vi "SVT STFT vs Time (Intensity).vi"(0 "scaled signal [EU]":waveform(dbl), 5 "FFT block size":i32=1024 min=1, 7 "window":T8(ring)=enum."Hanning", 9 "time segment":T7={"from [s]"=-1.0, "to [s]"=-1.0, "time increment"=100.0, "time increment units (%)"=enum."%"} {"time increment" format="%.2f"; "to [s]" format="%.2f"; "from [s]" format="%.2f"}, 11 "error in (no error)":errorcluster, 12 "dB On (T)":bool=TRUE, 13 "weighting":u16(ring) items=["Linear", "A-weighting", "B-weighting", "C-weighting"]) -> (4 "power spectra [dB EU]":dbl[][](array[numeric]) format="%.2f", 6 "unit label":string, 8 "f0 and delta f [Hz]":cluster{"f0":dbl, "delta f":dbl}={"f0"=0.0, "delta f"=0.0009765625} {"delta f" format="%.2f"; "f0" format="%.2f"}, 10 "t0 and delta t [s]":cluster{"t0":dbl, "delta t":dbl} {"delta t" format="%.2f"; "t0" format="%.2f"}, 14 "spectrum info":T1={"channel name"="", "description"="", "x-axis units"=0, "spectral info"={"spectrum type"=enum."Power [Magnitude^2]", "linear/dB"=enum."linear", "window"=0, "window size"=0, "FFT size"=0}, "engineering units"=0, "custom label"="", "dB reference [EU]"=0.0, "peak units"=enum."rms", "weighting filter"=0, "spectral density?"=FALSE, "unit label"="", "spectrum skewed?"=FALSE, "complimentary spectrum units"=enum."none"} {"x-axis units" items=["Time (s)"=0, "Frequency-CB (Hz)"=1, "Frequency-CPB (Hz)"=1248, "Frequency-Arbitrary (Hz)"=2357, "Quefrency (s)"=2, "Revolutions (rev)"=3, "Order"=4, "Speed (RPM)"=11, "Speed (rad/s)"=21, "Index"=65535]; "weighting filter" items=["Linear", "A-weighting", "B-weighting", "C-weighting", "ITU-R 468-4", "Dolby", "CCITT", "C-message", "Wb", "Wc", "Wd", "We", "Wf", "Wh", "Wj", "Wk", "Wm", "AES17 20 kHz lowpass", "AES17 40 kHz lowpass", "AES17 20 kHz highpass", "AES17 40 kHz highpass"]; "dB reference [EU]" format="%.2f"; "engineering units" items=["custom..."=0, "V"=1, "A"=21, "C"=30, "pC"=31, "s"=32, "-"=29, "Pa"=2, "N"=20, "g"=3, "m/s^2"=4, "m/s"=5, "m"=6, "mm/s"=12, "mm"=13, "micron/s"=14, "micron"=15, "in/s^2"=7, "in/s"=8, "in"=9, "mil/s"=10, "mil"=11, "rad/s^2"=16, "rad/s"=17, "rad"=18, "deg/s^2"=26, "deg/s"=27, "deg"=28, "RPM"=22, "cycle/s^2"=23, "Hz"=24, "cycle"=25, "strain"=19]; "spectral info"."window" items=["None "=0, "Hanning"=1, "Hamming"=2, "Blackman-Harris"=3, "Exact Blackman"=4, "Blackman"=5, "Flat Top"=6, "4 Term B-Harris "=7, "7 Term B-Harris"=8, "Low Sidelobe"=9, "Force - Exponential"=10, "Gaussian"=62]}, 15 "error out":errorcluster)   [LabVIEW 2017, in "SoundVib_Transient.lvlib"]
doc: "Performs a short-time Fourier transform (STFT) on <B>scaled signal [EU]</B> and returns the power spectrum, waterfall, or colormap at the various times you specify. Wire data to the <B>scaled signal [EU]</B> input to determine the polymorphic instance to use or manually select the instance."
uses:
  <vilib>/addons/Sound and Vibration/svt_Transients/SoundVib_Transient.lvlib
  <vilib>/addons/_NISVFA/_Shared subVIs/Controls/svc_Spectrum Info.ctl
  <vilib>/addons/_NISVFA/_Shared subVIs/Controls/svc_X-Axis Units.ctl
  <vilib>/addons/_NISVFA/_Shared subVIs/Controls/svc_Spectrum Type.ctl
  <vilib>/addons/_NISVFA/_Shared subVIs/Controls/svc_Engineering Units Text Ring.ctl
  <vilib>/addons/_NISVFA/_Shared subVIs/Controls/svc_Weighting Filter Text Ring.ctl
  <vilib>/addons/_NISVFA/_Shared subVIs/Controls/svc_Complimentary Spectrum Units.ctl
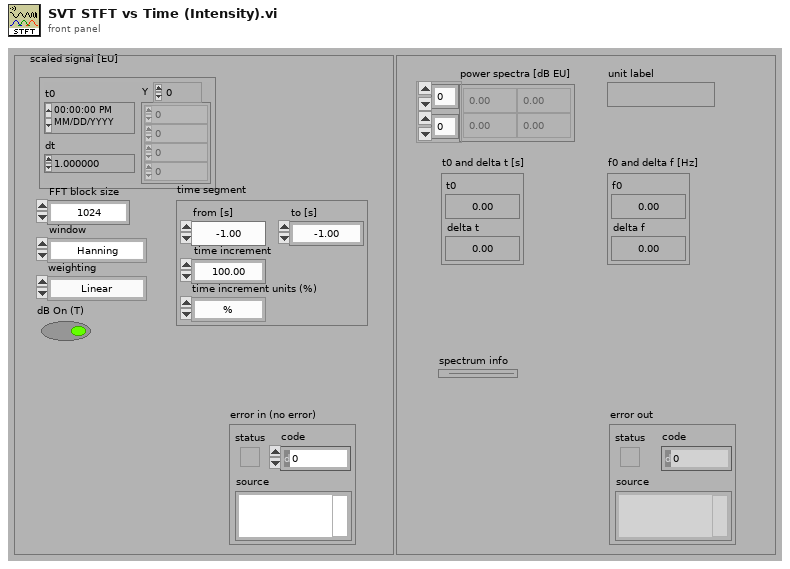
[diagram p1: front panel]
types:
  T1 = typedef "svc_Spectrum Info.ctl" = cluster{"channel name":string, "description":string, "x-axis units":T2, "spectral info":cluster{"spectrum type":T3, "linear/dB":enum16{"linear", "dB"}, "window":u16, "window size":i32, "FFT size":i32}, "engineering units":T4, "custom label":string, "dB reference [EU]":dbl, "peak units":enum16{"rms", "peak", "peak-peak"}, "weighting filter":T5, "spectral density?":bool, "unit label":string, "spectrum skewed?":bool, "complimentary spectrum units":T6}
  T2 = typedef "svc_X-Axis Units.ctl" = u16
  T3 = typedef "svc_Spectrum Type.ctl" = enum16{"FFT Spectrum [complex]", "Amplitude [Magnitude]", "Power [Magnitude^2]", "Cross Spectrum [complex]", "Frequency Response [Complex]"}
  T4 = typedef "svc_Engineering Units Text Ring.ctl" = u16
  T5 = typedef "svc_Weighting Filter Text Ring.ctl" = u16
  T6 = typedef "svc_Complimentary Spectrum Units.ctl" = enum16{"none", "radians", "degrees", "cycles", "imaginary"}
  T7 = cluster{"from [s]":dbl, "to [s]":dbl, "time increment":dbl, "time increment units (%)":enum16{"%", "s", "ms"}}
  T8 = enum16{"None ", "Hanning", "Hamming", "Blackman-Harris", "Exact Blackman", "Blackman", "Flat Top", "4 Term B-Harris ", "7 Term B-Harris", "Low Sidelobe"}
  T9 = cluster{"FFT block size":i32, "number of FFT":i32, "start index":i32, "increment":dbl}
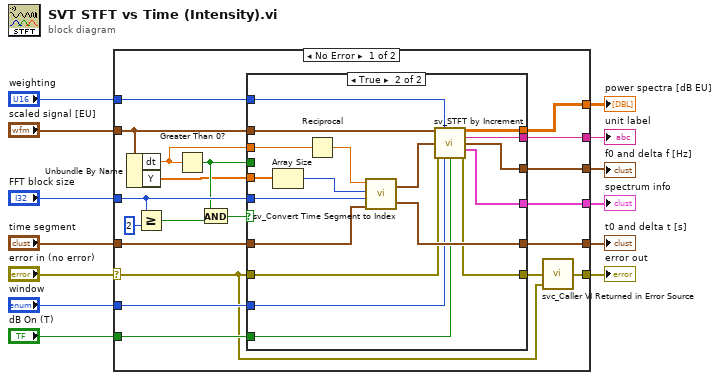
[diagram p0: block diagram]
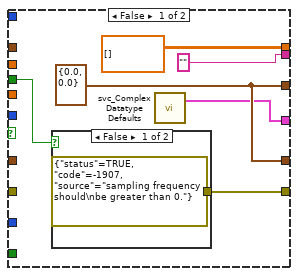
[diagram p2: hidden frame]
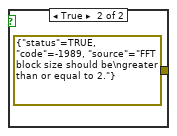
[diagram p3: hidden frame]
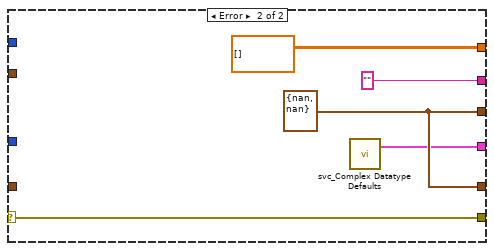
[diagram p4: hidden frame]
diagram:
  n1 = case shown="No Error" "error in (no error)" {
    selector: "error in (no error)" -> [w15 w64]
    tunnel: "dB On (T)" -> [w30 _]
    tunnel: "window" -> [w31 _]
    tunnel: "FFT block size" -> [w25 _]
    tunnel: "time segment" -> [w33 _]
    tunnel: "scaled signal [EU]" -> [w21 _]
    tunnel: [w22 w64] -> w7
    tunnel: [w27 "" ("unit label")] -> w6
    tunnel: [w32 w61] -> w5
    tunnel: [w28 dbl[][] [] ("power spectrum [EU^2 rms]")] -> w4
    tunnel: [w26 w61] -> w3
    tunnel: "weighting" -> [w29 _]
    tunnel: [w14 w60] -> w1
    frame No Error {
      n2 = Unbundle By Name(w21) -> ("dt"=w17:dbl, "Y"=w16:dbl[])
      n3 = Greater Or Equal?(x=w25, y=2) -> (x >= y?=w20:bool)
      n4 = Greater Than 0?(x=w17) -> (x > 0?=w18:bool)
      n5 = And(x=w18, y=w20) -> (x .and. y?=w19:bool)
      n6 = case shown="True" w19 {
        tunnel: w25 -> [_ w58]
        tunnel: w33 -> [_ w57]
        tunnel: [w36 w56] -> w32
        tunnel: w31 -> [_ w54]
        tunnel: w30 -> [_ w53]
        tunnel: w29 -> [_ w52]
        tunnel: [dbl[][] [] ("power spectra [dB EU]") w51] -> w28
        tunnel: ["" ("unit label") w50] -> w27
        tunnel: [w36 w43] -> w26
        tunnel: w21 -> [_ w49]
        tunnel: w15 -> [_ w47]
        tunnel: [w39 w46] -> w23
        tunnel: w18 -> [w35 _]
        tunnel: w17 -> [_ w45]
        tunnel: w16 -> [_ w44]
        tunnel: [w34 w42] -> w14
        frame False {
          w36 = cluster{"f0":dbl, "delta f":dbl} {"f0"=0.0, "delta f"=0.0} ("f0 and delta f [Hz]")
          n7 = case shown="False" w35 {
            tunnel: [errorcluster {"status"=TRUE, "code"=-1907, "source"="sampling frequency should\nbe greater than 0."} ("error out") errorcluster {"status"=TRUE, "code"=-1989, "source"="FFT block size should be\ngreater than or equal to 2."} ("error out")] -> w39
            frame False {
            }
            frame True {
            }
          }
          n8 = call <vilib>:"svc_Complex Datatype Defaults.vi"() -> ("dead spectrum info"=w34:T1)  [unwired: 11 in, 8 out]
        }
        frame True {
          n9 = Array Size(array=w44) -> (size(s)=w59:i32)
          n10 = Reciprocal(x=w45) -> (1/x=w48:dbl)
          n11 = call <vilib>:"sv_Convert Time Segment to Index.vi"("sampling frequency [Hz]"=w48, "array size"=w59, "FFT block size"=w58, "time segment"=w57) -> ("FFT info"=w55:T9, "to and delta t [s]"=w56:cluster{"to":dbl, "delta t":dbl})  [unwired: 1 in]
          n12 = call <vilib>:"sv_STFT by Increment.vi"("scaled signal [EU]"=w49, "weighting filter"=w52, "FFT info"=w55, "error in (no error)"=w47, "window"=w54, "dB On (T)"=w53) -> ("power spectra [dB EU]"=w51:dbl[][], "unit label"=w50:string, "f0 and delta f [Hz]"=w43:cluster{"f0":dbl, "delta f":dbl}, "spectrum info"=w42:T1, "error out"=w46:errorcluster)  [unwired: 5 in]
        }
      }
      n13 = call <vilib>:"svc_Caller VI Returned in Error Source.vi"("warning input to caller"=w15, "error in (no error)"=w23) -> ("error out"=w22:errorcluster)  [unwired: 3 in]
    }
    frame Error {
      w61 = cluster{"f0":dbl, "delta f":dbl} {"f0"=nan, "delta f"=nan} ("f0 and delta f [Hz]")
      n14 = call <vilib>:"svc_Complex Datatype Defaults.vi"() -> ("dead spectrum info"=w60:T1)  [unwired: 11 in, 8 out]
    }
  }
  "error out" <- w7
  "unit label" <- w6
  "f0 and delta f [Hz]" <- w3
  "t0 and delta t [s]" <- w5
  "power spectra [dB EU]" <- w4
  "spectrum info" <- w1
